vi "Publish Error.vi"(8 "error in (no error)":errorcluster, 11 "CS++DeviceActor in":refnum<class "CS++DeviceActor.lvclass">) -> (0 "error out":errorcluster, 3 "CS++DeviceActor out":refnum<class "CS++DeviceActor.lvclass">)   [LabVIEW 2012, in "CS++DeviceActor.lvlib" / "CS++DeviceActor.lvclass"]
doc: "Publish error info."
uses:
  CS++DeviceActor.lvclass
  Classes/CS++ProcessVariables/ProcessVariable/PV.lvclass
  <vilib>/Utility/error.llb/DialogType.ctl
  CS++DeviceActor.lvclass/CS++DeviceActor.ctl
  Classes/CS++ProcessVariables/PVConnection/PVConnection.lvclass
  Classes/CS++ProcessVariables/ProcessVariable/PV.lvclass/PV.ctl
  Classes/CS++ProcessVariables/ProcessVariable/Write Timestamp.vi
  Classes/CS++ProcessVariables/ProcessVariable/Write Quality.vi
  Classes/CS++ProcessVariables/ProcessVariable/Write status.vi
  Classes/CS++ProcessVariables/ProcessVariable/Write Data.vi
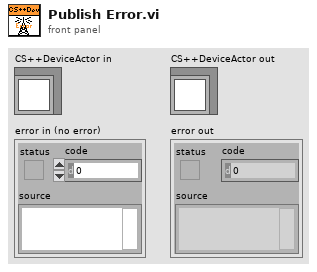
[diagram p1: front panel]
types:
  T1 = typedef "DialogType.ctl" = u16
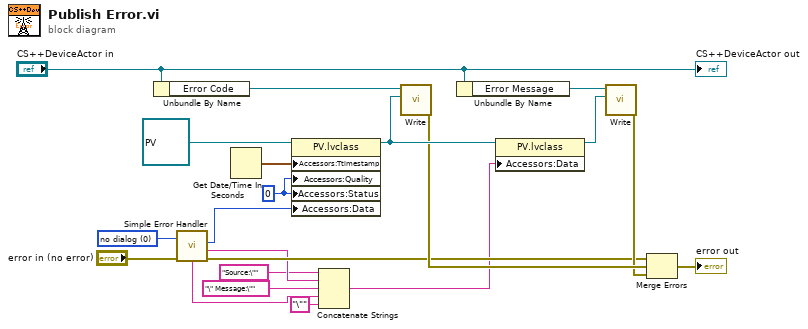
[diagram p0: block diagram]
diagram:
  w8 = T1 0 items=["no dialog", "OK message", "continue or stop message", "OK message + warnings", "continue/stop + warnings"] ("type of dialog (OK msg:1)")
  w11 = 0 ("Quality")
  n1 = Unbundle By Name("CS++DeviceActor in") -> ("Error Code"=w21:refnum<class "PVConnection.lvclass">)
  n2 = call <vilib>:"Simple Error Handler.vi"("type of dialog (OK msg:1)"=w8, "error in (no error)"="error in (no error)") -> ("code out"=w7:i32, "source out"=w6:string, "error out"=w9:errorcluster, "message"=w3:string)  [unwired: 3 in, 1 out]
  n3 = Get Date/Time In Seconds() -> (seconds since 1Jan1904=w19:timestamp)
  n4 = property class="PV.lvclass"(reference=refnum<class "PV.lvclass"> refnum ("CS++ProcessVariables.lvlib:PV.lvclass"), "Accessors:Ttimestamp"=w19, "Accessors:Quality"=w11, "Accessors:Status"=w11, "Accessors:Data"=w7) -> (reference out=w17:refnum<class "PV.lvclass">)  [unwired: 1 in, 1 out]
  n5 = Concatenate Strings("Source:\"" ("string"), w6, "\" Message:\"" ("string"), w3, "\"" ("string")) -> (w1:string)
  n6 = call-dynamic "Write.vi"("PV"=w17, "PVConnection in"=w21) -> ("error out"=w15:errorcluster)  [unwired: 8 in, 1 out]
  n7 = Unbundle By Name("CS++DeviceActor in") -> ("Error Message"=w18:refnum<class "PVConnection.lvclass">)
  n8 = property class="PV.lvclass"(reference=w17, "Accessors:Data"=w1) -> (reference out=w12:refnum<class "PV.lvclass">)  [unwired: 1 in, 1 out]
  n9 = call-dynamic "Write.vi"("PV"=w12, "PVConnection in"=w18) -> ("error out"=w14:errorcluster)  [unwired: 8 in, 1 out]
  n10 = Merge Errors(w9, w15, w14) -> (→"error out":errorcluster)
  "CS++DeviceActor out" <- "CS++DeviceActor in"
